vi "Convert-U64-to-String.vi"(8 "error in":errorcluster, 9 "Array (U64) in 2":u64[](array[numeric]) format="%.0x", 10 "Array (U64) in":u64[](array[numeric]) format="%.0x", 11 "Title":string="FIFO Dump") -> (0 "error out":errorcluster, 3 "String out":string)   [LabVIEW 2018]
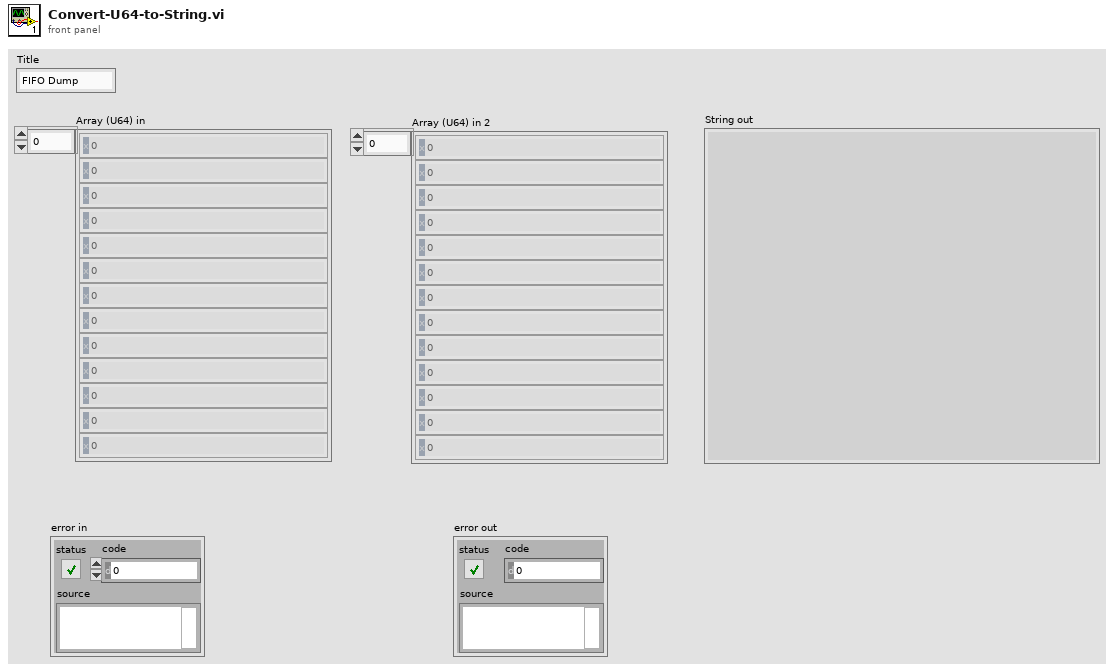
[diagram p1: front panel]
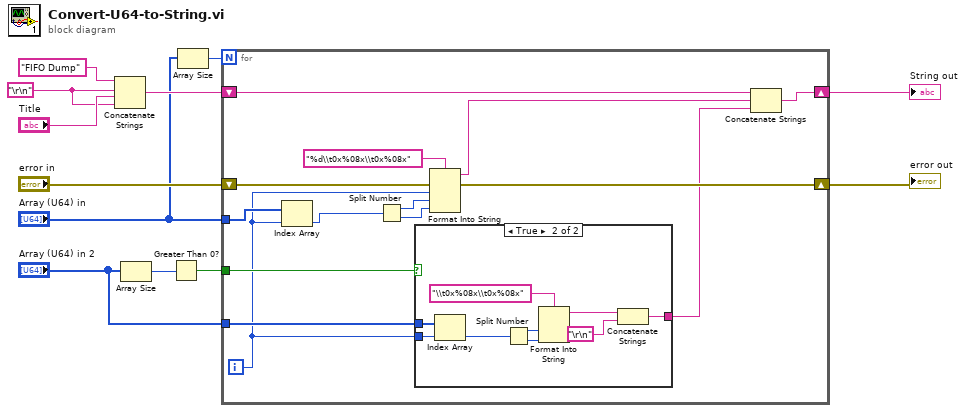
[diagram p0: block diagram]
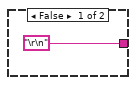
[diagram p2: hidden frame]
diagram:
  w8 = "\r\n"
  n1 = Concatenate Strings("FIFO Dump", w8, "Title", w8) -> (w10:string)
  n2 = Array Size(array="Array (U64) in 2") -> (size(s)=w3:i32)
  n3 = Greater Than 0?(x=w3) -> (x > 0?=w2:bool)
  n4 = Array Size(array="Array (U64) in") -> (size(s)=w5:i32)
  n5 = for {
    N: w5 -> [_]
    tunnel: "Array (U64) in" -> [w18]
    shift-right: [w23] -> w12
    shift-left: w10 -> [w25]
    shift-right: [w20] -> w7
    shift-left: "error in" -> [w19]
    tunnel: w2 -> [w16]
    tunnel: "Array (U64) in 2" -> [w15]
    i -> [w14]
    n6 = Index Array(array=w18, index=w14) -> (element=w17:u64)
    n7 = Split Number(x=w17) -> (hi(x)=w22:u32, lo(x)=w21:u32)
    n8 = case shown="True" w16 {
      tunnel: w15 -> [_ w36]
      tunnel: w14 -> [_ w35]
      tunnel: ["\r\n" w30] -> w13
      frame False {
      }
      frame True {
        n9 = Index Array(array=w36, index=w35) -> (element=w32:u64)
        n10 = Split Number(x=w32) -> (hi(x)=w34:u32, lo(x)=w33:u32)
        n11 = Format Into String(format string="\\t0x%08x\\t0x%08x", w34, w33) -> (resulting string=w28:string)  [unwired: 2 in, 1 out]
        n12 = Concatenate Strings(w28, "\r\n") -> (w30:string)
      }
    }
    n13 = Format Into String(format string="%d\\t0x%08x\\t0x%08x", error in=w19, w14, w22, w21) -> (resulting string=w24:string, error out=w20:errorcluster)  [unwired: 1 in]
    n14 = Concatenate Strings(w25, w24, w13) -> (w23:string)
  }
  "String out" <- w12
  "error out" <- w7
